vi "SailSetSuggestions.vi"() -> ()   [LabVIEW 2012]
doc: "Eric Schneider and Bonnie Ishiguro\nSpring 2014\n\nReturns suggestions for the sail positions (0-1) based on the current state of the boat. This outputs a number of suggestions, which are blended in the arbiter in Act.\n\nInputs: relative wind angle, degree of luffing, rudder force, the direction of the boat, and the desired direction of the boat"
panel:
  in  "DesiredHeading":dbl
  in  "RobotHeading":dbl
  in  "RudderForce":dbl
  in  "DegreeOfLuffing":dbl
  in  "RelativeWindAngle":dbl
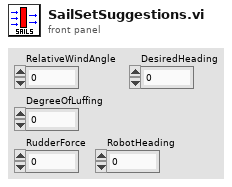
[diagram p1: front panel]
types:
  T1 = enum16{"Straight", "Turning", "Approach Maneuver", "Cross Wind (Tack)", "Cross Wind (Gybe)", "Turtle Mode", ""}
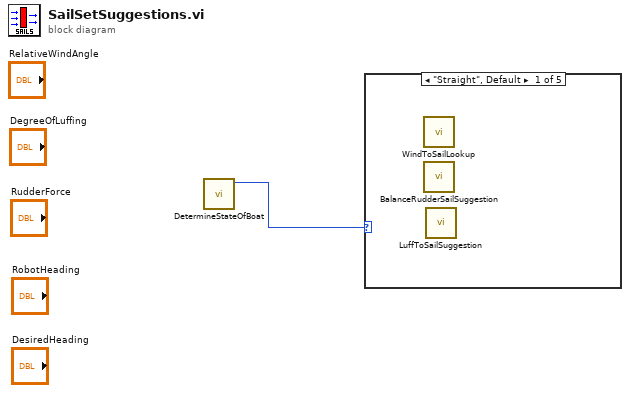
[diagram p0: block diagram]
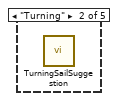
[diagram p2: hidden frame]
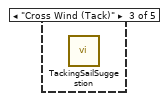
[diagram p3: hidden frame]
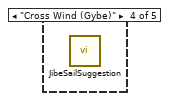
[diagram p4: hidden frame]
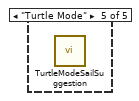
[diagram p5: hidden frame]
diagram:
  n1 = call "DetermineStateOfBoat.vi"() -> ("StateOfBoat"=w1:T1)  [unwired: 9 in, 1 out]
  n2 = case shown="\"Straight\", Default" w1 {
    frame "Straight", Default {
      n3 = call "WindToSailLookup.vi"() -> ()  [unwired: 12 in]
      n4 = call "BalanceRudderSailSuggestion.vi"() -> ()  [unwired: 11 in, 1 out]
      n5 = call "LuffToSailSuggestion.vi"() -> ()  [unwired: 10 in, 2 out]
    }
    frame "Turning" {
      n6 = call "TurningSailSuggestion.vi"() -> ()  [unwired: 12 in]
    }
    frame "Cross Wind (Tack)" {
      n7 = call "TackingSailSuggestion.vi"() -> ()  [unwired: 9 in, 3 out]
    }
    frame "Cross Wind (Gybe)" {
      n8 = call "JibeSailSuggestion.vi"() -> ()  [unwired: 9 in, 3 out]
    }
    frame "Turtle Mode" {
      n9 = call "TurtleModeSailSuggestion.vi"() -> ()  [unwired: 12 in]
    }
  }
